vi "Check_FailMessage.vi"(9 "All_Result":bool[](array[boolean]), 10 "测试数据":refnum<vi>, 11 "ListBox输入":refnum<vi>) -> ()   [LabVIEW 2018]
panel:
  out "数组":string[](array[string])
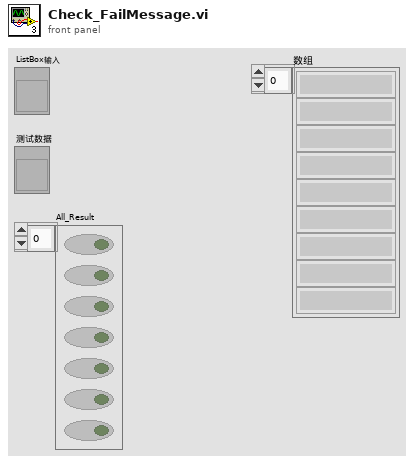
[diagram p1: front panel]
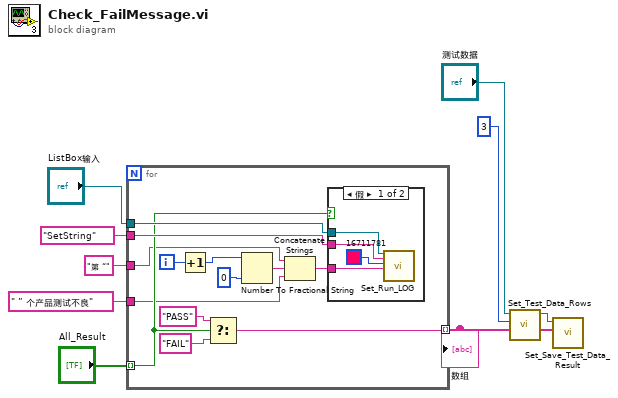
[diagram p0: block diagram]
diagram:
  n1 = for {
    tunnel: "All_Result" -> [w17] mode=indexing
    tunnel: [w21] -> w1 mode=indexing
    tunnel: "SetString" ("组合框") -> [w20]
    tunnel: "第 “" -> [w12]
    tunnel: "ListBox输入" -> [w18]
    tunnel: " ” 个产品测试不良" -> [w11]
    i -> [w19]
    n2 = Increment(x=w19) -> (x+1=w14:i32)
    n3 = Select(t="PASS" ("字符串"), s=w17, f="FAIL" ("字符串")) -> (s? t:f=w21:string)
    n4 = Number To Fractional String(number=w14, precision (6)=i16 0 ("精度(6)")) -> (F-format string=w15:string)  [unwired: 2 in]
    n5 = Concatenate Strings(w12, w15, w11) -> (w16:string)
    n6 = case shown="假" w17 {
      tunnel: w20 -> [w27 _]
      tunnel: w16 -> [w26 _]
      tunnel: w18 -> [w25 _]
      frame False {
        n7 = call "Set_Run_LOG.vi"("列表框 3"=w25, "组合框"=w27, "颜色盒"=u32 16711781, "字符串"=w26) -> ()  [unwired: 14 in, 2 out]
      }
      frame True {
      }
    }
  }
  "数组" <- w1
  n8 = call "Set_Test_Data_Rows.vi"("输入行数据"=w1, "索引 (行)"=3, "测试数据 2"="测试数据") -> ("数组"=w5:string[], "引用输出"=w4:refnum<vi>)  [unwired: 7 in]
  n9 = call "Set_Save_Test_Data_Result.vi"("Result Arry"=w5, "测试数据 2"=w4) -> ()  [unwired: 9 in, 1 out]
